vi "Write Fetch Room Sizes Msg.vi"(10 "Guest Manager UI.lvlib:Fetch Room Sizes Msg.lvclass":refnum<class "Fetch Room Sizes Msg.lvclass">, 11 "Guest Manager UI in":refnum<class "Guest Manager UI.lvclass">) -> (3 "Guest Manager UI out":refnum<class "Guest Manager UI.lvclass">)   [LabVIEW 2023, in "Guest Manager UI.lvlib" / "Guest Manager UI.lvclass"]
uses:
  Guest Manager UI.lvclass
  Guest Manager UI Messages/Fetch Room Sizes Msg/Fetch Room Sizes Msg.lvclass
  Guest Manager UI.lvclass/Guest Manager UI.ctl
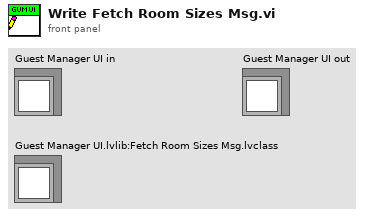
[diagram p1: front panel]
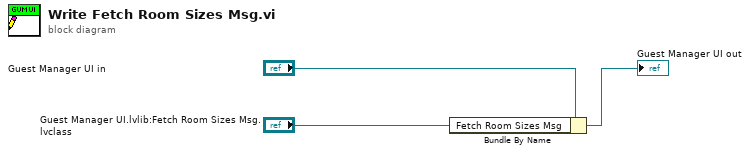
[diagram p0: block diagram]
diagram:
  n1 = Bundle By Name(cluster="Guest Manager UI in", "Fetch Room Sizes Msg"="Guest Manager UI.lvlib:Fetch Room Sizes Msg.lvclass") -> (→"Guest Manager UI out":refnum<class "Guest Manager UI.lvclass">)
